vi "test_Swap Slot.vi"(8 "error in (no error)":errorcluster, 11 "TestCase in":refnum<class "Scan Engine Scripting API Custom Device Unit Tests.lvclass">) -> (0 "error out":errorcluster, 3 "TestCase out":refnum<class "Scan Engine Scripting API Custom Device Unit Tests.lvclass">)   [LabVIEW 2017, in "Scan Engine Scripting API Custom Device Unit Tests.lvclass"]
uses:
  Scan Engine Scripting API Custom Device Unit Tests.lvclass
  Scan Engine Scripting API Custom Device Unit Tests.lvclass/Scan Engine Scripting API Custom Device Unit Tests.ctl
  Type Defs/Main Settings.ctl
  Type Defs/Local Chassis Settings.ctl
  Scripting/Modules/NI 9224/NI 9224.lvclass
  C:/dev/niveristand-scan-engine-ethercat-custom-device/Custom Device Source/Scripting/Modules/Module/Module.lvclass
  Scripting/Modules/Module/Module.lvclass
  Scripting/Modules/Utility/Shared Properties/Conversion Time.ctl
  03383bdb-f803-46da-afce-439191e079c9.vi
  e351be74-a324-4f38-992a-dbd26274029f.vi
  22ffbf48-dcc3-43bb-9d82-770fbbdd10ca.vi
  d9141057-35de-479b-b1a6-8872e0885cb5.vi
  Utility/Set Error.vi
  <vilib>/Utility/error.llb/Clear Errors.vi
  Modules.lvlibp/SD Module/SD Module.lvclass
  C:/dev/niveristand-scan-engine-ethercat-custom-device/Custom Device Source/Modules.lvlibp/RSI Module/RSI Module.lvclass
  Scripting/Modules/NI 9228/NI 9228.lvclass
  Modules.lvlibp/RSI Module/Read Module Page Property.vi
  Modules.lvlibp/RSI Module/Read Model.vi
  Scripting/Utility/Convert Module Model to Module Class.vi
  Modules.lvlibp/SD Module/Read DIO mode.vi
  Modules.lvlibp/RSI Module/Read Channels.vi
  Scripting/Utility/Convert to DI Module.vi
  Scripting/Utility/Convert to DO Module.vi
  Scripting/Utility/Convert to CI PWM Module.vi
  Scripting/Utility/Convert to CDO Module.vi
  Scripting/Utility/Convert to PWM Module.vi
  Globals/Error Strings.vi
  Scripting/Utility/Convert to AI Vrms Module.vi
  Scripting/Utility/Convert to AI Module.vi
  Modules.lvlibp/9224/9224.lvclass
  <vilib>/addons/_JKI Toolkits/VI Tester/TestCase.llb/TestCase.lvclass
  Scripting/Scan Engine Scripting.lvlib
  Scan Engine Custom Device.lvlib
  C:/Program Files (x86)/National Instruments/LabVIEW 2017/vi.lib/addons/_JKI Toolkits/VI Tester/TestCase.llb/TestCase.lvclass
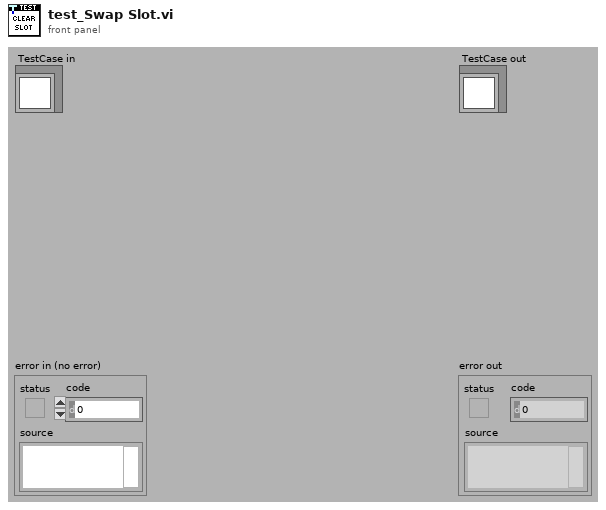
[diagram p1: front panel]
types:
  T1 = typedef "Scan Engine Custom Device.lvlib/Main Settings.ctl" = cluster{"sync to scan":bool, "scan engine decimation":u16, "delay after FPGA load (s)":u16}
  T2 = typedef "Scan Engine Custom Device.lvlib/Local Chassis Settings.ctl" = cluster{"name":string, "number of slots":i32}
  T3 = typedef "Scan Engine Scripting.lvlib/Conversion Time.ctl" = enum16{"High Speed (1k S/s)", "Medium Speed (100 S/s)", "Medium Resolution (50/60Hz Rejection - 12 S/s)", "High Resolution (50/60Hz Rejection - 2 S/s)"}
  T4 = typedef "Custom Device API.lvlib/Custom Device Item Ref.ctl" = u64
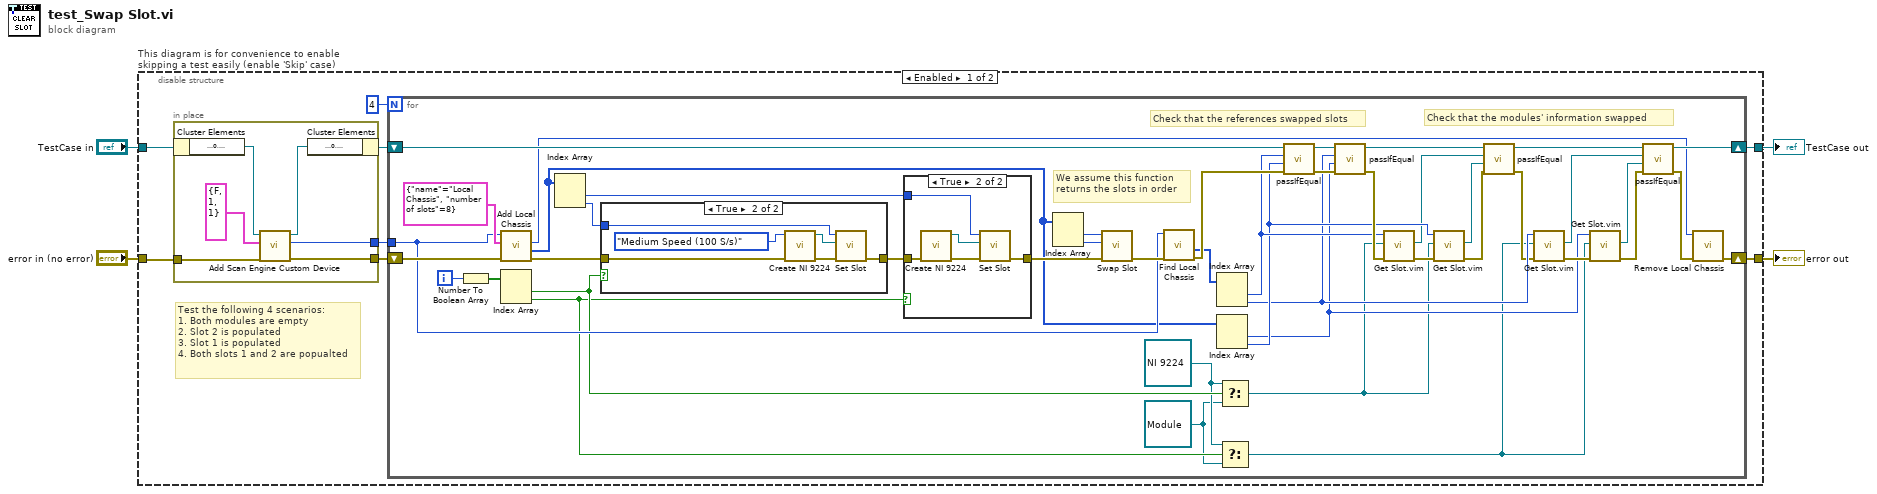
[diagram p0: block diagram]
diagram:
  n1 = disable-structure "This diagram is for convenience to enable skipping a test easily (enable 'Skip' case)" shown="Enabled" {
    disable-tunnel: "TestCase in" -> [w9 w80]
    disable-tunnel: [w7 w78] -> w1
    disable-tunnel: [w6 w79] -> w3
    disable-tunnel: "error in (no error)" -> [w10 w77]
    frame Enabled {
      # "Test the following 4 scenarios:\n1. Both modules are empty\n2. Slot 2 is populated\n3. Slot 1 is populated\n4. Both slots 1 and 2 are popualted"
      n2 = in-place {
        in-place-border: [w18] -> w12
        in-place-border: [w17] -> w11
        in-place-border: w10 -> [w15]
        n3 = in-place-cluster #1(w9) -> ("target ref"=w14:refnum<k24>)
        n4 = call "Add Scan Engine Custom Device.vi"("error in"=w15, "settings"=T1 {"sync to scan"=FALSE, "scan engine decimation"=1, "delay after FPGA load (s)"=1}, "target in"=w14) -> ("error out"=w17:errorcluster, "scan engine custom device ref"=w18:T4, "target out"=w13:refnum<k24>)  [unwired: 6 in]
        n5 = in-place-cluster #1("target ref"=w13) -> (w8:refnum<class "Scan Engine Scripting API Custom Device Unit Tests.lvclass">)
      }
      n6 = for {
        N: 4 -> [_]
        tunnel: w12 -> [w50]
        shift-right: [w20] -> w6
        shift-left: w11 -> [w63]
        shift-right: [w32] -> w7
        shift-left: w8 -> [w48]
        i -> [w60]
        w22 = refnum<class "Module.lvclass"> refnum ("Scan Engine Scripting.lvlib:Module.lvclass")
        w23 = refnum<class "NI 9224.lvclass"> refnum ("NI 9224 out")
        # "Check that the modules' information swapped"
        # "Check that the references swapped slots"
        # "We assume this function returns the slots in order"
        n7 = Number To Boolean Array(number=w60) -> (Boolean array=w59:bool[])
        n8 = call "Add Local Chassis.vi"("error in"=w63, "settings"=T2 {"name"="Local Chassis", "number of slots"=8}, "scan engine custom device ref in"=w50) -> ("error out"=w58:errorcluster, "slot refs"=w45:T4[], "local chassis ref"=w19:T4)  [unwired: 4 in, 2 out]
        n9 = Index Array(array=w59) -> (element #1=w27:bool, element #2=w26:bool)  [unwired: 2 in]
        n10 = Index Array(array=w45) -> (element #1=w56:T4, element #2=w57:T4)  [unwired: 2 in]
        n11 = case shown="True" w27 {
          tunnel: w58 -> [w70 w75]
          tunnel: w57 -> [_ w72]
          tunnel: [w70 w74] -> w55
          frame False {
          }
          frame True {
            n12 = call "Create NI 9224.vi"("error in"=w75, "conversion time"=Conversion_Time."Medium Speed (100 S/s)") -> ("error out"=w76:errorcluster, "NI 9224 out"=w73:refnum<class "NI 9224.lvclass">)  [unwired: 8 in]
            n13 = call "Set Slot.vi"("error in"=w76, "module"=w73, "slot ref in"=w72) -> ("error out"=w74:errorcluster)  [unwired: 7 in, 1 out]
          }
        }
        n14 = case shown="True" w26 {
          tunnel: w55 -> [w64 w68]
          tunnel: w56 -> [_ w65]
          tunnel: [w64 w67] -> w54
          frame False {
          }
          frame True {
            n15 = call "Create NI 9224.vi"("error in"=w68) -> ("error out"=w69:errorcluster, "NI 9224 out"=w66:refnum<class "NI 9224.lvclass">)  [unwired: 9 in]
            n16 = call "Set Slot.vi"("error in"=w69, "module"=w66, "slot ref in"=w65) -> ("error out"=w67:errorcluster)  [unwired: 7 in, 1 out]
          }
        }
        n17 = Index Array(array=w45) -> (element #1=w52:T4, element #2=w53:T4)  [unwired: 2 in]
        n18 = call "Swap Slot.vi"("error in"=w54, "slot 2 ref in"=w53, "slot 1 ref in"=w52) -> ("error out"=w51:errorcluster)  [unwired: 6 in, 2 out]
        n19 = call "Find Local Chassis.vi"("error in"=w51, "scan engine custom device ref in"=w50) -> ("error out"=w61:errorcluster, "slots refs"=w46:T4[])  [unwired: 4 in, 4 out]
        n20 = Index Array(array=w46) -> (element #1=w40:T4, element #2=w38:T4)  [unwired: 2 in]
        n21 = Index Array(array=w45) -> (element #1=w37:T4, element #2=w39:T4)  [unwired: 2 in]
        n22 = Select(t=w23, s=w27, f=w22) -> (s? t:f=w25:refnum<class "Module.lvclass">)
        n23 = Select(t=w23, s=w26, f=w22) -> (s? t:f=w24:refnum<class "Module.lvclass">)
        n24 = call-dynamic "passIfEqual.vi"("error in (no error)"=w61, "y"=w39, "x"=w40, "TestCase in"=w48) -> ("error out"=w49:errorcluster, "TestCase out"=w47:refnum<class "Scan Engine Scripting API Custom Device Unit Tests.lvclass">)  [unwired: 6 in]
        n25 = call-dynamic "passIfEqual.vi"("error in (no error)"=w49, "y"=w37, "x"=w38, "TestCase in"=w47) -> ("error out"=w44:errorcluster, "TestCase out"=w33:refnum<class "Scan Engine Scripting API Custom Device Unit Tests.lvclass">)  [unwired: 6 in]
        n26 = call "Get Slot.vim"("error in"=w44, "module in"=w25, "slot ref in"=w40) -> ("error out"=w43:errorcluster, "module"=w29:refnum<class "Module.lvclass">)  [unwired: 5 in, 2 out]
        n27 = call "Get Slot.vim"("error in"=w43, "module in"=w25, "slot ref in"=w39) -> ("error out"=w34:errorcluster, "module"=w28:refnum<class "Module.lvclass">)  [unwired: 5 in, 2 out]
        n28 = call-dynamic "passIfEqual.vi"("error in (no error)"=w34, "y"=w28, "x"=w29, "TestCase in"=w33) -> ("error out"=w35:errorcluster, "TestCase out"=w41:refnum<class "Scan Engine Scripting API Custom Device Unit Tests.lvclass">)  [unwired: 6 in]
        n29 = call "Get Slot.vim"("error in"=w35, "module in"=w24, "slot ref in"=w38) -> ("error out"=w42:errorcluster, "module"=w30:refnum<class "Module.lvclass">)  [unwired: 5 in, 2 out]
        n30 = call "Get Slot.vim"("error in"=w42, "module in"=w24, "slot ref in"=w37) -> ("error out"=w36:errorcluster, "module"=w31:refnum<class "Module.lvclass">)  [unwired: 5 in, 2 out]
        n31 = call-dynamic "passIfEqual.vi"("error in (no error)"=w36, "y"=w31, "x"=w30, "TestCase in"=w41) -> ("error out"=w21:errorcluster, "TestCase out"=w32:refnum<class "Scan Engine Scripting API Custom Device Unit Tests.lvclass">)  [unwired: 6 in]
        n32 = call "Remove Local Chassis.vi"("error in"=w21, "local chassis ref"=w19) -> ("error out"=w20:errorcluster)  [unwired: 9 in]
      }
    }
    frame Disabled {
      # "skip test result while test is under development"
      n33 = call <vilib>:"skip.vi"("error in (no error)"=w77, "TestCase in"=w80) -> ("error out"=w79:errorcluster, "TestCase out"=w78:refnum<class "Scan Engine Scripting API Custom Device Unit Tests.lvclass">)  [unwired: 8 in]
    }
  }
  "error out" <- w3
  "TestCase out" <- w1
